vi "Build Map.vi"(5 "Walls":cluster{"Y":dbl, "X":dbl}[](array[cluster]), 6 "Objects bottom cords":T1(array[cluster]), 7 "Robot":cluster{"Y":dbl, "X":dbl, "Bearing":dbl}) -> (1 "Updated Corners":cluster{"Col":i16, "Row":i16}[](array[cluster]), 2 "Updated Map":i8[][](array[numeric]), 3 "Robot in map":cluster{"Col":i16, "Row":i16})   [LabVIEW 2009]
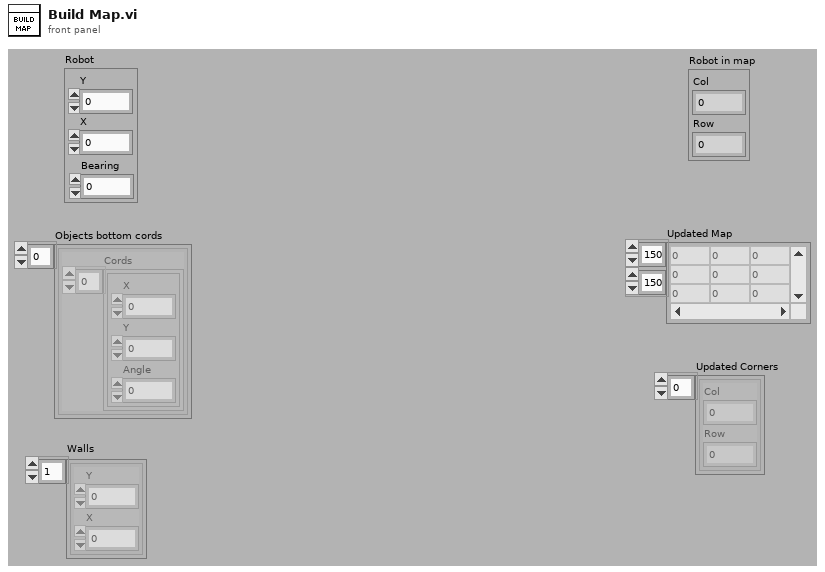
[diagram p1: front panel]
types:
  T1 = cluster{"Cords":cluster{"X":dbl, "Y":dbl, "Angle":dbl}[]}[]
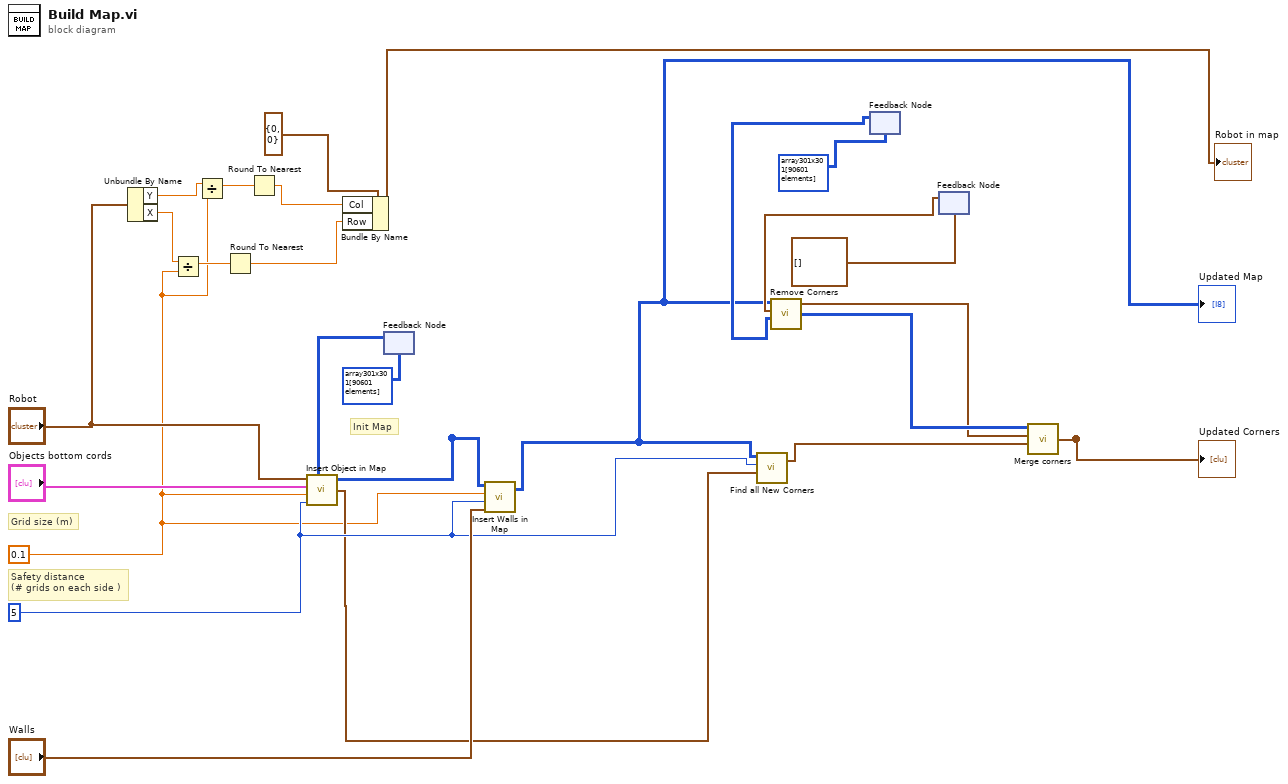
[diagram p0: block diagram]
diagram:
  w13 = 5
  w5 = 0.1
  # "Init Map"
  # "Safety distance \n(# grids on each side )"
  # "Grid size (m)"
  n1 = Unbundle By Name("Robot") -> ("Y"=w6:dbl, "X"=w8:dbl)
  n2 = Divide(x=w8, y=w5) -> (x/y=w10:dbl)
  n3 = Divide(x=w6, y=w5) -> (x/y=w7:dbl)
  n4 = Round To Nearest(number=w10) -> (nearest integer value=w1:dbl)
  n5 = Round To Nearest(number=w7) -> (nearest integer value=w2:dbl)
  n6 = Bundle By Name(cluster=cluster{"Col":i16, "Row":i16} {"Col"=0, "Row"=0} ("Robot cluster"), "Col"=w2, "Row"=w1) -> (→"Robot in map":cluster{"Col":i16, "Row":i16})
  n7 = feedback #1(i8[][] array301x301[90601 elements] ("matrix")) -> (w17:i8[][])
  n8 = call "Insert Object in Map.vi"("Robot"="Robot", "Map"=w17, "Objects bottom cords"="Objects bottom cords", "Grid size (m)"=w5, "# safety grids"=w13) -> ("Updated Map"=w15:i8[][], "Points"=w12:cluster{"Col":i16, "Row":i16}[])  [unwired: 2 in]
  n9 = call "Insert Walls in Map.vi"("Map"=w15, "Grid size"=w5, "# safety grids"=w13, "Walls"="Walls") -> ("Updated Map"=w14:i8[][])  [unwired: 2 in]
  "Updated Map" <- w14
  n10 = call "Find all New Corners.vi"("Points"=w12, "# safety grids"=w13, "Updated Map"=w14) -> ("Corners"=w11:cluster{"Col":i16, "Row":i16}[])  [unwired: 2 in]
  n11 = feedback #2(i8[][] array301x301[90601 elements] ("Updated Corners Matrix")) -> (w24:i8[][])
  n12 = feedback #3(cluster{"Col":i16, "Row":i16}[] [] ("New old corners")) -> (w21:cluster{"Col":i16, "Row":i16}[])
  n13 = call "Remove Corners.vi"("Old Corners Matrix"=w24, "Old corners"=w21, "Updated Map"=w14) -> ("Updated Corners Matrix"=w27:i8[][], "New old corners"=w26:cluster{"Col":i16, "Row":i16}[])  [unwired: 2 in]
  n14 = call "Merge corners.vi"("New Corners"=w11, "Old corners"=w26, "Corners Matrix"=w27) -> ("Updated Corners"=w22:cluster{"Col":i16, "Row":i16}[], "Updated Corners Matrix"=w25:i8[][])  [unwired: 2 in]
  "Updated Corners" <- w22
